vi "Get Exchanges To Date.vi"(8 "error in (no error)":errorcluster caption="entrée d'erreur (pas d'erreur)", 10 "Date":timestamp, 11 "Exchanges en entrée":refnum<class "Exchanges.lvclass"> caption="DNL_LabVIEW Object in") -> (0 "error out":errorcluster caption="sortie d'erreur", 1 "Min Date":timestamp, 2 "Exchanges to Date":T1[](array[typedef]), 3 "Exchanges en sortie":refnum<class "Exchanges.lvclass"> caption="DNL_LabVIEW Object out")   [LabVIEW 2012, in "Exchanges.lvclass"]
uses:
  Exchanges.lvclass
  Exchange/Exchange Parameters.ctl
  Exchange/Exchange Type Enum.ctl
  controls/Currencies.ctl
  Exchange/Exchange.lvclass
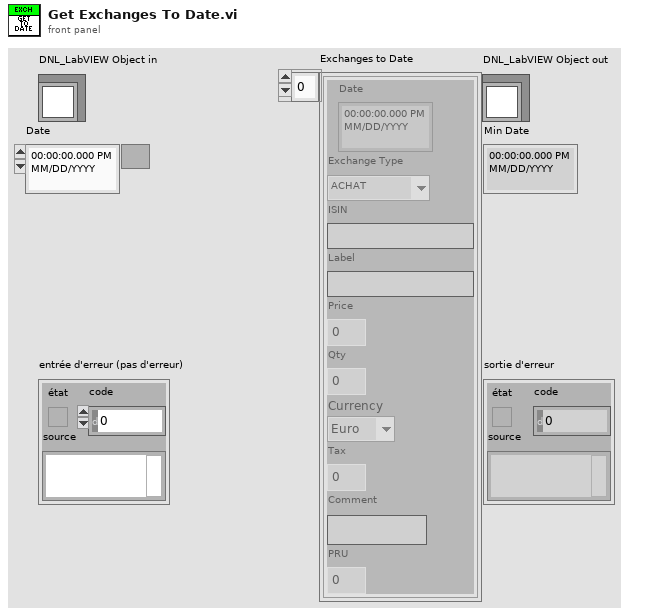
[diagram p1: front panel]
types:
  T1 = typedef "Exchange Parameters.ctl" = cluster{"Date":timestamp, "Exchange Type":T2, "ISIN":string, "Label":string, "Price":dbl, "Qty":dbl, "Currency":T3, "Tax":dbl, "Comment":string, "PRU":dbl}
  T2 = typedef "Exchange.lvclass/Exchange Type Enum.ctl" = enum16{"ACHAT", "VENTE"}
  T3 = typedef "Currencies.ctl" = enum16{"Euro", "Dollar", "Yen", "RIM", "CHF"}
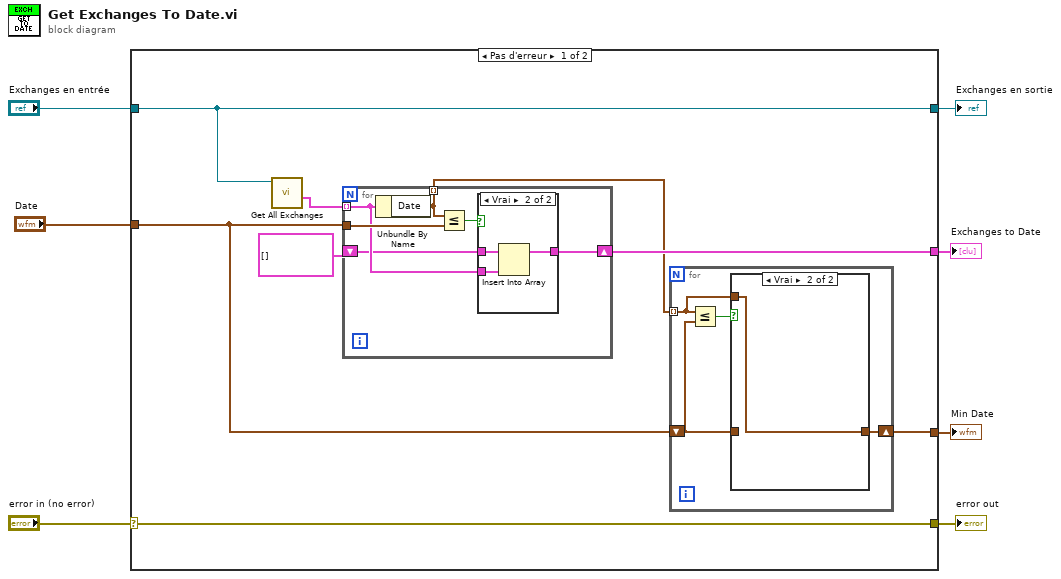
[diagram p0: block diagram]
diagram:
  n1 = case shown="Pas d'erreur" "error in (no error)" {
    selector: "error in (no error)" -> [w15 w34]
    tunnel: [w15 w34] -> w6
    tunnel: [w12 w33] -> w4
    tunnel: "Exchanges en entrée" -> [w12 w33]
    tunnel: [w11 _] -> w3
    tunnel: [w9 w32] -> w2
    tunnel: "Date" -> [w8 w32]
    frame No Error {
      n2 = call "Get All Exchanges.vi"("Exchanges en entrée"=w12) -> ("Exchanges"=w14:T1[])  [unwired: 6 in, 4 out]
      n3 = for {
        tunnel: w14 -> [w25] mode=indexing
        tunnel: w8 -> [w27]
        shift-right: [w24] -> w11
        shift-left: T1[] [] -> [w23]
        tunnel: [w22] -> w10 mode=indexing
        n4 = Unbundle By Name(w25) -> ("Date"=w22:timestamp)
        n5 = Less Or Equal?(x=w22, y=w27) -> (x <= y?=w26:bool)
        n6 = case shown="Vrai" w26 {
          tunnel: w25 -> [_ w31]
          tunnel: [w28 w30] -> w24
          tunnel: w23 -> [w28 w29]
          frame False {
          }
          frame True {
            n7 = Insert Into Array(array=w29, new element=w31) -> (w30:T1[])  [unwired: 1 in]
          }
        }
      }
      n8 = for {
        tunnel: w10 -> [w18] mode=indexing
        shift-right: [w17] -> w9
        shift-left: w8 -> [w16]
        n9 = Less Or Equal?(x=w18, y=w16) -> (x <= y?=w19:bool)
        n10 = case shown="Vrai" w19 {
          tunnel: w18 -> [_ w21]
          tunnel: [w20 w21] -> w17
          tunnel: w16 -> [w20 _]
          frame False {
          }
          frame True {
          }
        }
      }
    }
    frame Error {
    }
  }
  "error out" <- w6
  "Exchanges en sortie" <- w4
  "Exchanges to Date" <- w3
  "Min Date" <- w2
